vi "phincalculator.vi"() -> ()   [LabVIEW 2015]
panel:
  out "Phi(n)":i32
  in  "Numeric":i32 caption="Ingrese un \nnumero para\n calcular phi(n)"
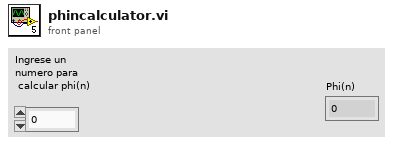
[diagram p1: front panel]
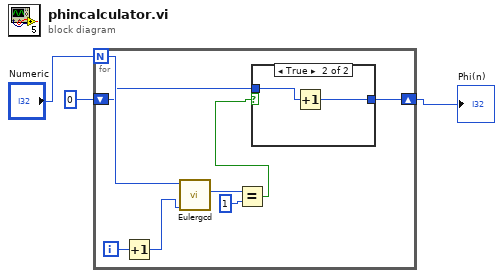
[diagram p0: block diagram]
diagram:
  n1 = for {
    N: "Numeric" -> [w11]
    shift-right: [w6] -> w1
    shift-left: 0 -> [w7]
    i -> [w5]
    n2 = Increment(x=w5) -> (x+1=w4:i32)
    n3 = call "Eulergcd.vi"("b"=w4, "a"=w11) -> ("r"=w10:i32)  [unwired: 9 in]
    n4 = Equal?(x=w10, y=1) -> (x = y?=w8:bool)
    n5 = case shown="True" w8 {
      tunnel: w7 -> [w12 w14]
      tunnel: [w12 w13] -> w6
      frame False {
      }
      frame True {
        n6 = Increment(x=w14) -> (x+1=w13:i32)
      }
    }
  }
  "Phi(n)" <- w1
